vi "CalcAngleError.vi"(9 "DesiredAngle":dbl format="%#_13g", 10 "ActualAngle":dbl format="%#_13g") -> (2 "Error":dbl)   [LabVIEW 2013]
doc: "Calculates the difference between the actual angle and the desired angle. The returned error is on the interval [-180, 180]. (A positive number means the robot must rotate counterclockwise, a negative number means the robot must rotate clockwise.)"
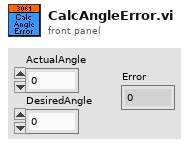
[diagram p1: front panel]
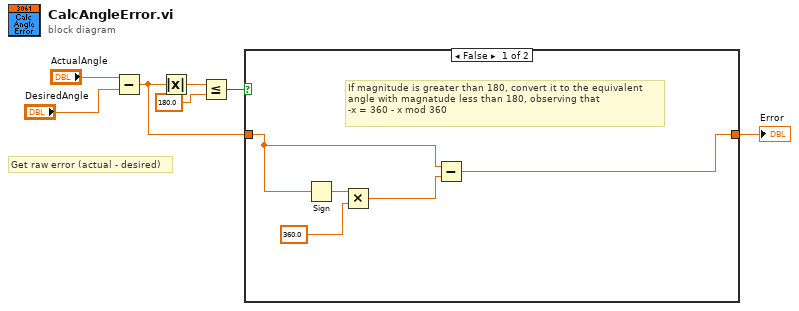
[diagram p0: block diagram]
diagram:
  # "Get raw error (actual - desired)"
  n1 = Subtract(x="ActualAngle", y="DesiredAngle") -> (x-y=w4:dbl)
  n2 = Absolute Value(x=w4) -> (abs(x)=w7:dbl)
  n3 = Less Or Equal?(x=w7, y=180.0) -> (x <= y?=w5:bool)
  n4 = case shown="False" w5 {
    tunnel: w4 -> [w9 w13]
    tunnel: [w8 w13] -> w3
    frame False {
      # "If magnitude is greater than 180, convert it to the equivalent\nangle with magnatude less than 180, observing that\n-x = 360 - x mod 360"
      n5 = Sign(1:w9) -> (0:w12:dbl)
      n6 = Multiply(x=w12, y=360.0) -> (x*y=w10:dbl)
      n7 = Subtract(x=w9, y=w10) -> (x-y=w8:dbl)
    }
    frame True {
      # "If magnitude of difference is less than 180, no processing needed"
    }
  }
  "Error" <- w3
